vi "Vision Processing.vi"(4 "error in (no error)":errorcluster, 6 "CameraDevRef":T1) -> ()   [LabVIEW 2011]
uses:
  <vilib>/Rock Robotics/WPI/Camera/WPI_CameraDevRef.ctl
  Robot Global Data.vi
  <vilib>/vision/NI_Vision_Development_Module.lvlib
panel:
  in  "Run Calculations":bool
  out "Raw Turret":dbl
  out "Target X Coord":dbl
  out "Target Distance":dbl
  out "Target Y Coord":dbl
  out "Distance Array":dbl[](array[numeric])
  in  "Scaler":dbl=0.85
  in  "Lower Speed Limit":dbl=0.05
  out "Number of Rectangles Visible":dbl
  out "Y Position Array":dbl[](array[numeric])
  out "X Position Array":dbl[](array[numeric])
  in  "View":bool
  out "Target Info":T2(array[cluster])
  in  "Area Size Limit":i32=444
  in  "Particle Count Limit":i32=8
  in  "Score Limits":T3={"Rect Coverage"=76.0, "Aspect Ratio"=40.0, "X Edge Strength"=40.0, "Y Edge Strength"=60.0}
  in  "Processing":enum32{"Color", "Intensity", "Intensity Open"}(tab)=enum."Intensity Open"
  in  "Luminance":i32=255
  in  "Saturation":i32=255
  in  "Hue":i32(knob)=65 scale=0.0..255.0
  in  "Margins":cluster{"Hue":i32, "Sat":i32, "Lum":i32}={"Hue"=20, "Sat"=27, "Lum"=30} {"Sat" scale=0.0..40.0; "Lum" scale=0.0..40.0; "Hue" scale=0.0..40.0}
  in  "Range":cluster{"Lower value":sgl, "Upper value":sgl}={"Lower value"=150.0, "Upper value"=255.0} {"Lower value" scale=0.0..255.0; "Upper value" scale=0.0..255.0}
  in  "Range":cluster{"Lower value":sgl, "Upper value":sgl}={"Lower value"=123.804344, "Upper value"=255.0} {"Lower value" scale=0.0..255.0; "Upper value" scale=0.0..255.0}
  in  "View":bool
  out "Processed Image":T4(plugin-control)
  out "Original Image":T4(plugin-control)
  # "Instructions:\nProcessing the reflective tape that is illuminated by a ring light can be based\non color or light intensity.\nParticles within the image are scored by rectangle coverage, aspect ratio, and\nfor being hollow with a bold edge. A particle is considered a target if all scores\nare above the score limits. Particles can be annotated -- surrounded by\na rectangle and scores drawn to the left .\nTo control the number of particles being scored, use the count limit and the size\nlimit."
  # "To debug, Enable using the View button.\nFor color processing, you can click in the image to select the color for processing."
  # "Enable by clicking the View button.\nGreen scores are above the limit, orange are below. Inner/outer rect\nindicates all passed."
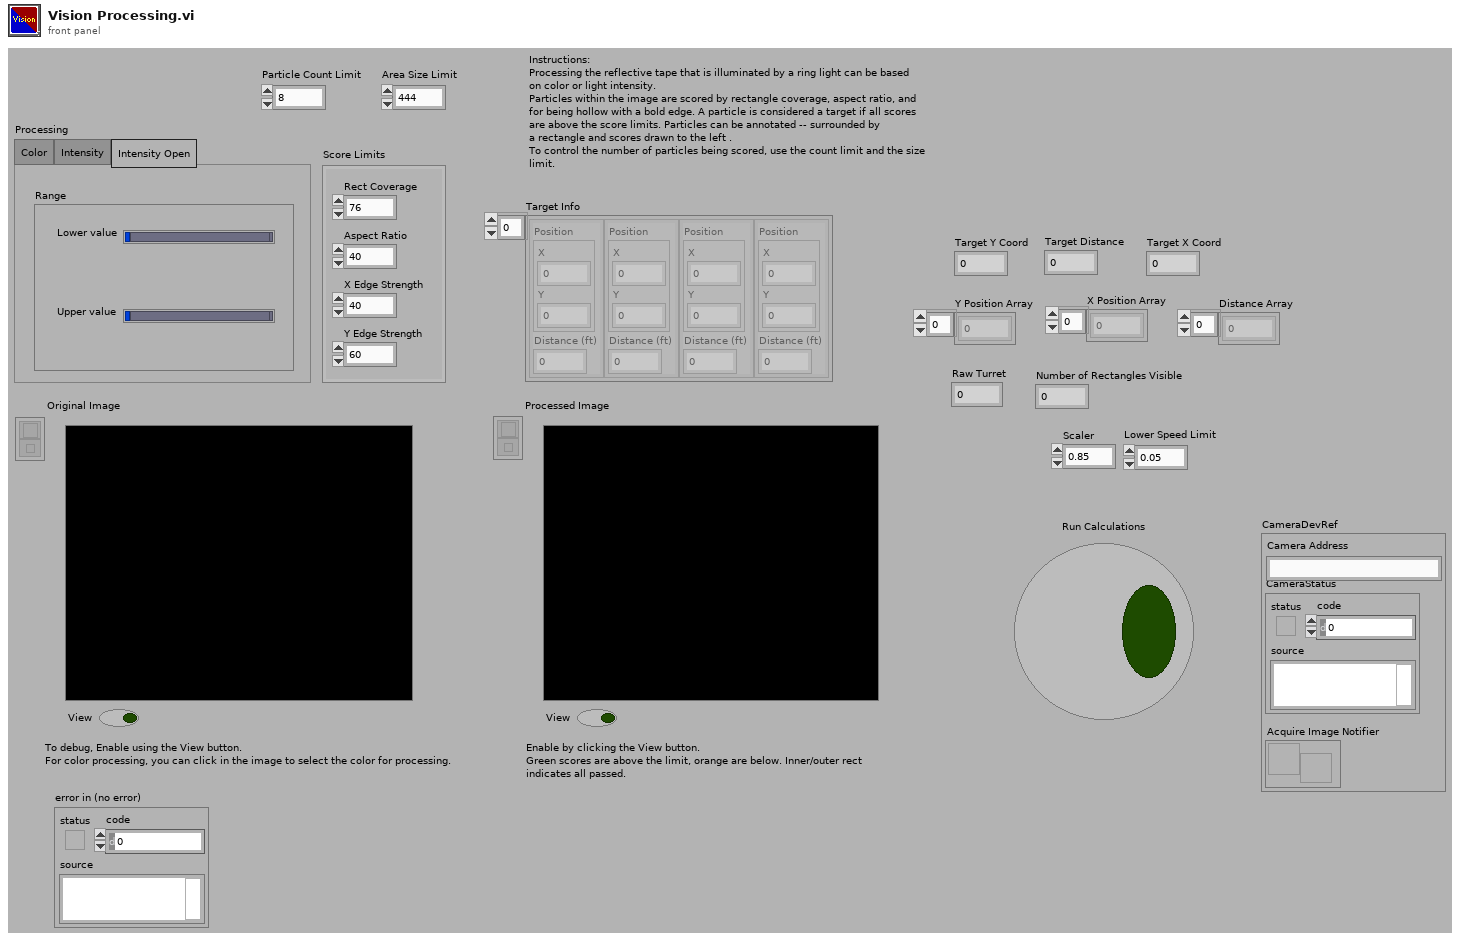
[diagram p1: front panel]
types:
  T1 = typedef "WPI_CameraDevRef.ctl" = cluster{"Camera Address":string, "CameraStatus":errorcluster, "Acquire Image Notifier":refnum<notifier>}
  T2 = cluster{"Position":cluster{"X":dbl, "Y":dbl}, "Distance (ft)":dbl}[]
  T3 = cluster{"Rect Coverage":dbl, "Aspect Ratio":dbl, "X Edge Strength":dbl, "Y Edge Strength":dbl}
  T4 = typedef "IMAQ Image.ctl" = refnum<image>
  T5 = typedef "Image Type" = u32
  T6 = enum32{"AutoM", "Close", "Dilate", "Erode", "Gradient", "Gradient out", "Gradient in", "Hit miss", "Open", "PClose", "POpen", "Thick", "Thin"}
  T7 = typedef "WPI_CameraImageSize.ctl" = enum16{"640x480", "320x240", "160x120"}
  T8 = cluster{"fps":i32, "compression":i32, "Image Size":T7}
  T9 = cluster{cluster{"Left":dbl, "Top":dbl, "Right":dbl, "Bottom":dbl}, dbl[]}[]
  T10 = cluster{"Left":dbl, "Top":dbl, "Right":dbl, "Bottom":dbl}
  T11 = cluster{"Target Center (-1 to 1)":cluster{"X":dbl, "Y":dbl}, "Distance (ft)":dbl}
  T12 = cluster{"Target Center (-1 to 1)":cluster{"X":dbl, "Y":dbl}, "Distance (ft)":dbl}[]
  T13 = typedef "WPI_JoystickDevRef.ctl" = cluster{"Device":T14}
  T14 = typedef "WPI_JoystickDeviceEnum.ctl" = enum16{"USB 1", "USB 2", "USB 3", "USB 4", "Kinect 1", "Kinect 2"}
  T15 = typedef "WPI_JoystickButtonState.ctl" = cluster{"Button 1":bool, "Button 2":bool, "Button 3":bool, "Button 4":bool, "Button 5":bool, "Button 6":bool, "Button 7":bool, "Button 8":bool, "Button 9":bool, "Button 10":bool, "Button 11":bool, "Button 12":bool}
  T16 = cluster{"axis 1 (x)":dbl, "axis 2 (y)":dbl, "axis 3 (throttle)":dbl, "axis 4":dbl, "axis 5":dbl, "axis 6":dbl}
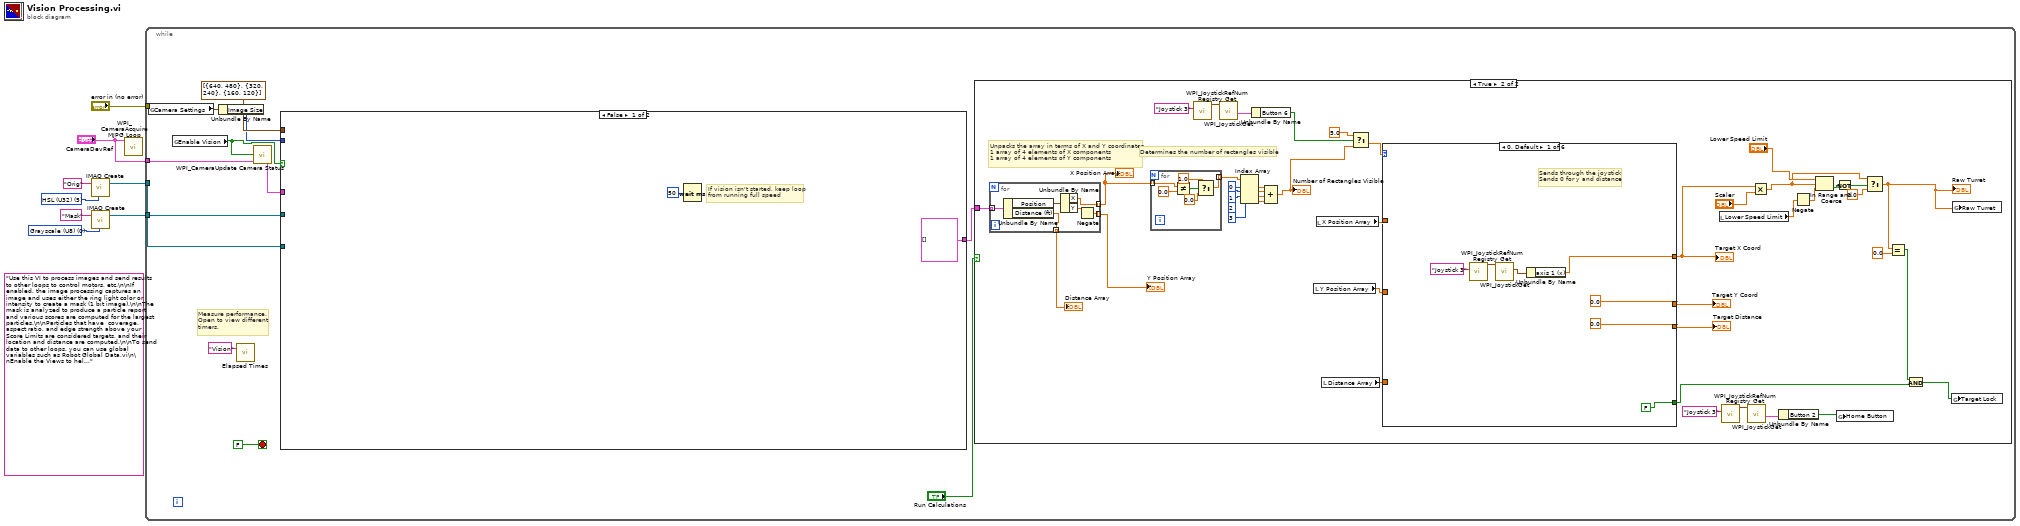
[diagram p0: block diagram]
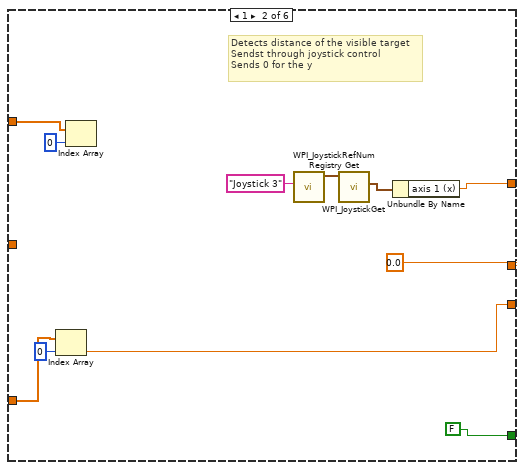
[diagram p3: hidden frame]
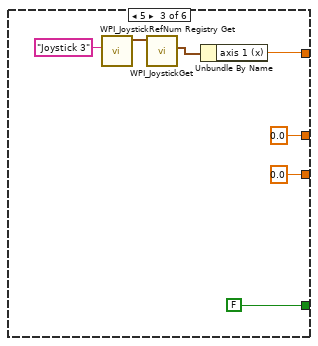
[diagram p4: hidden frame]
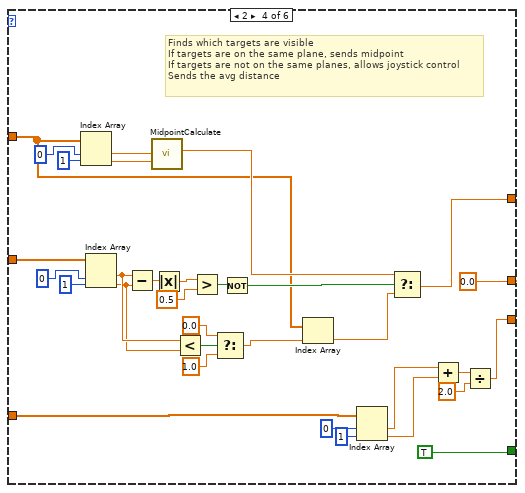
[diagram p5: hidden frame]
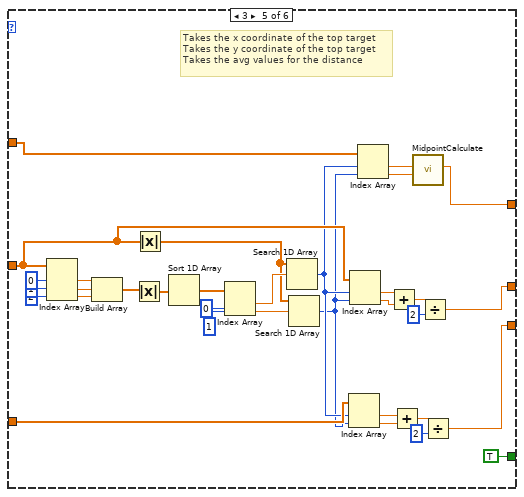
[diagram p6: hidden frame]
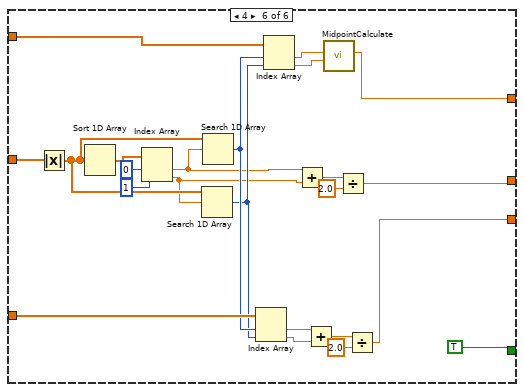
[diagram p7: hidden frame]
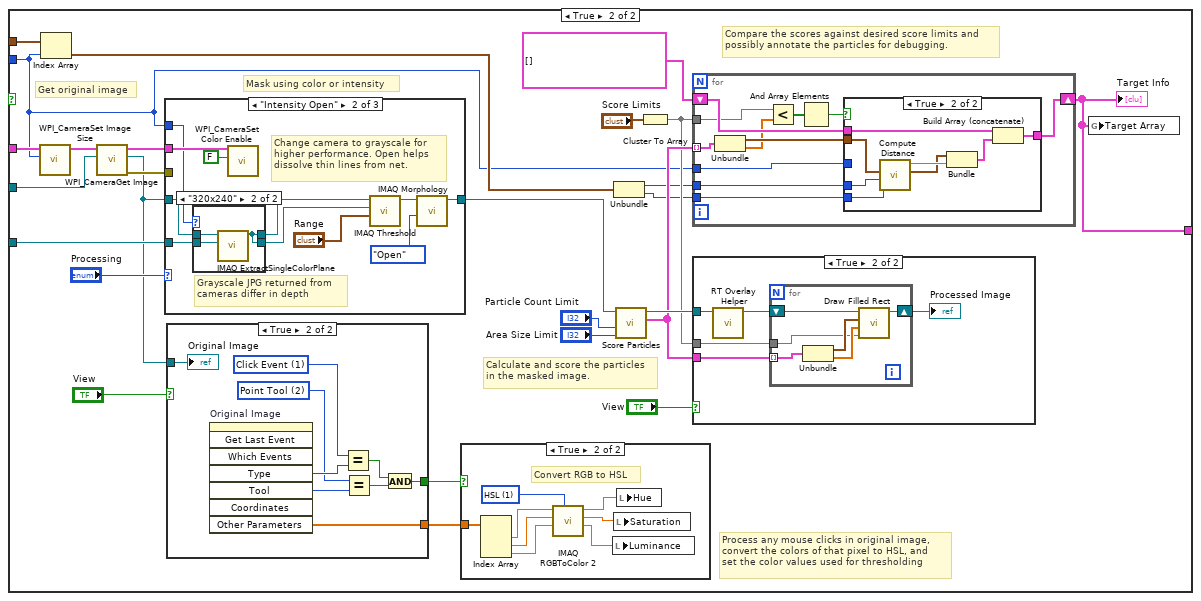
[diagram p8: hidden frame]
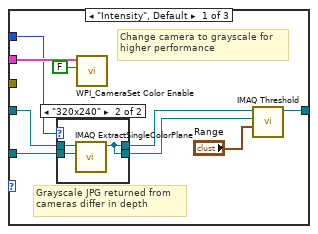
[diagram p10: hidden frame]
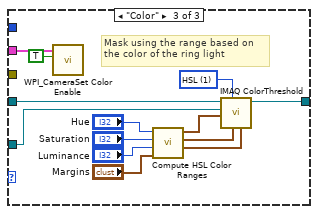
[diagram p13: hidden frame]
diagram:
  w3 = T5 0 items=["Grayscale (U8)", "Grayscale (I16)", "Grayscale (SGL)", "Complex (CSG)", "RGB (U32)", "HSL (U32)", "RGB (U64)", "Grayscale (U16)"] ("Image Type")
  (unwired) "Use this VI to process images and send results to other loops to control motors, etc.\n\nIf enabled, the image processing captures an image and uses either the ring light color or intensity to create a mask (1 bit image).\n\nThe mask is analyzed to produce a particle report and various scores are computed for the largest particles.\n\nParticles that have  coverage, aspect ratio, and edge strength above your Score Limits are considered targets, and their location and distance are computed.\n\nTo send data to other loops, you can use global variables such as Robot Global Data.vi\n\nEnable the Views to help debug color settings. Disable the View to speed up processing."
  w7 = T5 5 items=["Grayscale (U8)", "Grayscale (I16)", "Grayscale (SGL)", "Complex (CSG)", "RGB (U32)", "HSL (U32)", "RGB (U64)", "Grayscale (U16)"] ("Image Type")
  n1 = call "IMAQ Create"("Image Name"="Orig", "Image Type"=w7) -> ("New Image"=w6:T4)  [unwired: 2 in, 2 out]
  n2 = call "IMAQ Create"("Image Name"="Mask", "Image Type"=w3) -> ("New Image"=w1:T4)  [unwired: 2 in, 2 out]
  n3 = call <vilib>:"WPI_CameraAcquire MJPG Loop.vi"("CameraDevRef"="CameraDevRef") -> ()  [unwired: 11 in]
  n4 = while {
    tunnel: w6 -> [w19]
    tunnel: "CameraDevRef" -> [w18]
    tunnel: "error in (no error)" -> [_]
    tunnel: w1 -> [w14]
    stop <- FALSE stop-if-true
    # "Measure performance.\nOpen to view different\ntimers."
    n5 = global read "Robot Global Data.vi" "Camera Settings"() -> (w12:T8)
    n6 = global read "Robot Global Data.vi" "Enable Vision"() -> (w16:bool)
    n7 = Unbundle By Name(w12) -> ("Image Size"=w11:T7)
    n8 = call "Elapsed Times.vi"("Call Name"="Vision") -> ()  [unwired: 2 in, 1 out]
    n9 = call <vilib>:"WPI_CameraUpdate Camera Status.vi"("CameraDevRef In"=w18, "Enable Vision"=w16) -> ("CameraDevRef Out"=w17:T1)  [unwired: 3 in]
    n10 = case shown="False" w16 {
      tunnel: w19 -> [_ w207]
      tunnel: w17 -> [_ w203]
      tunnel: w14 -> [_ w194]
      tunnel: cluster{i32, i32}[] [{640, 480}, {320, 240}, {160, 120}] -> [_ w198]
      tunnel: w11 -> [_ w191]
      tunnel: [T2 [] w192] -> w10
      frame False {
        # "If vision isn't started, keep loop\nfrom running full speed"
        n11 = Wait (ms)(milliseconds to wait=u32 50) -> ()  [unwired: 1 out]
      }
      frame True {
        # "Compare the scores against desired score limits and\npossibly annotate the particles for debugging."
        # "Process any mouse clicks in original image,\nconvert the colors of that pixel to HSL, and\nset the color values used for thresholding"
        # "Calculate and score the particles\nin the masked image."
        # "Mask using color or intensity"
        # "Get original image"
        n12 = call <vilib>:"WPI_CameraSet Image Size.vi"("Image Size"=w191, "CameraDevRef"=w203) -> ("CameraDevRef Out"=w204:T1)  [unwired: 8 in, 1 out]
        n13 = Index Array(array=w198, index=w191) -> (element=w195:cluster{i32, i32})
        n14 = call <vilib>:"WPI_CameraGet Image.vi"("Image"=w207, "CameraDevRef"=w204) -> ("error out"=w205:errorcluster, "Image Out"=w193:T4, "CameraDevRef Out"=w206:T1)  [unwired: 7 in]
        n15 = case shown="\"Intensity Open\"" "Processing" {
          tunnel: w193 -> [w229 w241 w267]
          tunnel: [w232 w246 w266] -> w201
          tunnel: w206 -> [w230 w244 w257]
          tunnel: w205 -> [_ _ _]
          tunnel: w194 -> [w228 w242 w255]
          tunnel: w191 -> [w227 w243 _]
          frame "Intensity", Default {
            # "Grayscale JPG returned from\ncameras differ in depth"
            # "Change camera to grayscale for\nhigher performance"
            n16 = case shown="\"320x240\"" w227 {
              tunnel: w229 -> [w235 w238]
              tunnel: w228 -> [w234 w237]
              tunnel: [w235 w236] -> w226
              tunnel: [w234 w236] -> w225
              frame "640x480", Default {
              }
              frame "320x240" {
                n17 = call "IMAQ ExtractSingleColorPlane"("Image Dst"=w237, "Image Src"=w238) -> ("Image Dst Out"=w236:T4)  [unwired: 8 in, 1 out]
              }
            }
            n18 = call <vilib>:"WPI_CameraSet Color Enable.vi"("Color Enabled"=FALSE, "CameraDevRef"=w230) -> ()  [unwired: 8 in, 2 out]
            n19 = call "IMAQ Threshold"("Range"="Range", "Image Dst"=w225, "Image Src"=w226) -> ("Image Dst Out"=w232:T4)  [unwired: 3 in, 5 out]
          }
          frame "Intensity Open" {
            # "Grayscale JPG returned from\ncameras differ in depth"
            # "Change camera to grayscale for\nhigher performance. Open helps\ndissolve thin lines from net."
            n20 = case shown="\"320x240\"" w243 {
              tunnel: w241 -> [w251 w254]
              tunnel: w242 -> [w250 w253]
              tunnel: [w251 w252] -> w240
              tunnel: [w250 w252] -> w239
              frame "640x480", Default {
              }
              frame "320x240" {
                n21 = call "IMAQ ExtractSingleColorPlane"("Image Dst"=w253, "Image Src"=w254) -> ("Image Dst Out"=w252:T4)  [unwired: 8 in, 1 out]
              }
            }
            n22 = call <vilib>:"WPI_CameraSet Color Enable.vi"("Color Enabled"=FALSE, "CameraDevRef"=w244) -> ()  [unwired: 8 in, 2 out]
            n23 = call "IMAQ Threshold"("Range"="Range", "Image Dst"=w239, "Image Src"=w240) -> ("Image Dst Out"=w247:T4)  [unwired: 3 in, 5 out]
            n24 = call "IMAQ Morphology"("Operation"=T6."Open", "Image Src"=w247) -> ("Image Dst Out"=w246:T4)  [unwired: 8 in, 1 out]
          }
          frame "Color" {
            w265 = u16 1 items=["RGB", "HSL", "HSV", "HSI"] ("Color Mode")
            # "Mask using the range based on\nthe color of the ring light"
            n25 = call <vilib>:"WPI_CameraSet Color Enable.vi"("Color Enabled"=TRUE, "CameraDevRef"=w257) -> ()  [unwired: 8 in, 2 out]
            n26 = call "Compute HSL Color Ranges.vi"("Margins"="Margins", "Luminance"="Luminance", "Saturation"="Saturation", "Hue"="Hue") -> ("Lum Range"=w262:cluster{i32, i32}, "Sat Range"=w263:cluster{i32, i32}, "Hue Range"=w264:cluster{i32, i32})  [unwired: 5 in]
            n27 = call "IMAQ ColorThreshold"("Blue or Luma or Val or Inten Range"=w262, "Green or Sat Range"=w263, "Color Mode"=w265, "Red or Hue Range"=w264, "Image Dst"=w255, "Image Src"=w267) -> ("Image Dst Out"=w266:T4)  [unwired: 4 in, 1 out]
          }
        }
        n28 = case shown="True" "View" {
          tunnel: w193 -> [_ w287]
          tunnel: [_ w282] -> w200
          tunnel: [_ w279] -> w199
          frame False {
          }
          frame True {
            w280 = 2 items=["None", "Selection Tool", "Point Tool", "Line Tool", "Rectangle Tool", "Oval Tool", "Polygon Tool", "ClosedFreehandTool", "Annulus Tool", "Rotated Rectangle Tool", "Zoom Tool", "Pan Tool", "Polyline Tool", "Freehand Tool"] ("Tool")
            w281 = 1 items=["No Event"=0, "Click Event"=1, "Draw Event"=2, "Size Event"=4, "Scroll Event"=5, "Double Click Event"=8] ("Type")
            n29 = invoke on="Original Image" class="ImageControl" method="Get Last Event"() -> ("Type"=w283:i32, "Tool"=w286:i32, "Other Parameters"=w279:sgl[])  [unwired: 8 in, 5 out]
            n30 = Equal?(x=w281, y=w283) -> (x = y?=w284:bool)
            n31 = Equal?(x=w280, y=w286) -> (x = y?=w285:bool)
            n32 = And(x=w284, y=w285) -> (x .and. y?=w282:bool)
            "Original Image" <- w287
          }
        }
        n33 = case shown="True" w200 {
          tunnel: w199 -> [_ w224]
          frame False {
          }
          frame True {
            w223 = u16 1 items=["RGB", "HSL", "HSV", "HSI", "CIE L*a*b*", "CIE XYZ"] ("Color Mode")
            # "Convert RGB to HSL"
            n34 = Index Array(array=w224) -> (element #1=w222:sgl, element #2=w220:sgl, element #3=w218:sgl)  [unwired: 3 in]
            n35 = call "IMAQ RGBToColor 2"("Color Mode"=w223, "Blue value"=w218, "Green value"=w220, "Red value"=w222) -> ("Blue or Luma or Val or Inten or Z or b*value"=w217:dbl, "Green or Sat or Y or a* value"=w219:dbl, "Red or Hue or X or L* value"=w221:dbl)  [unwired: 4 in, 1 out]
            n36 = local write "Luminance"(w217) -> ()
            n37 = local write "Saturation"(w219) -> ()
            n38 = local write "Hue"(w221) -> ()
          }
        }
        n39 = Unbundle(w195) -> (w197:i32, w196:i32)
        n40 = call "Score Particles.vi"("Area Size Limit"="Area Size Limit", "Particle Count Limit"="Particle Count Limit", "Image Refnum in"=w201) -> ("Scored Particle Info"=w212:T9, "Image Refnum out"=w215:T4)  [unwired: 7 in]
        n41 = Cluster To Array(cluster="Score Limits") -> (array=w210:dbl[])
        n42 = for {
          shift-right: [w297] -> w192
          shift-left: T2 [] -> [w298]
          tunnel: w197 -> [w296]
          tunnel: w212 -> [w294] mode=indexing
          tunnel: w210 -> [w289]
          tunnel: w191 -> [w293]
          tunnel: w196 -> [w288]
          n43 = Unbundle(w294) -> (w295:T10, w290:dbl[])
          n44 = Less?(x=w289, y=w290) -> (x < y?=w292:bool[])
          n45 = And Array Elements(Boolean array=w292) -> (logical AND=w291:bool)
          n46 = case shown="True" w291 {
            tunnel: w298 -> [w299 w307]
            tunnel: [w299 w306] -> w297
            tunnel: w295 -> [_ w302]
            tunnel: w296 -> [_ w304]
            tunnel: w293 -> [_ _]
            tunnel: w288 -> [_ w301]
            frame False {
            }
            frame True {
              n47 = call "Compute Distance.vi"("Y Image Resolution"=w301, "X Image Resolution"=w304, "Bounding Box"=w302) -> ("Target Center (-1 to 1)"=w300:cluster{"X":dbl, "Y":dbl}, "Distance (ft)"=w303:dbl)  [unwired: 7 in]
              n48 = Bundle("Target Center (-1 to 1)"=w300, "Distance (ft)"=w303) -> (w305:T11)  [unwired: 1 in]
              n49 = Build Array (concatenate)(w307, w305) -> (w306:T12)
            }
          }
        }
        "Target Info" <- w192
        n50 = case shown="True" "View" {
          tunnel: w215 -> [_ w269]
          tunnel: w212 -> [_ w271]
          tunnel: w210 -> [_ w270]
          frame False {
          }
          frame True {
            n51 = call "RT Overlay Helper.vi"("Refnum in"=w269) -> ("Refnum out"=w272:T4)  [unwired: 10 in]
            n52 = for {
              shift-right: [w277] -> w268
              shift-left: w272 -> [w278]
              tunnel: w271 -> [w274] mode=indexing
              tunnel: w270 -> [w273]
              n53 = Unbundle(w274) -> (w275:T10, w276:dbl[])
              n54 = call "Draw Filled Rect.vi"("Limits"=w273, "Scores"=w276, "Bounding Box"=w275, "image in"=w278) -> ("image out"=w277:T4)  [unwired: 7 in]
            }
            "Processed Image" <- w268
          }
        }
        n55 = global write "Robot Global Data.vi" "Target Array"(w192) -> ()
      }
    }
    n56 = case shown="True" "Run Calculations" {
      tunnel: w10 -> [_ w35]
      frame False {
      }
      frame True {
        # "Determines the number of rectangles visible"
        # "Unpacks the array in terms of X and Y coordinates\n1 array of 4 elements of X components\n1 array of 4 elements of Y components"
        n57 = for {
          tunnel: [w186] -> w36 mode=indexing
          tunnel: [w187] -> w46 mode=indexing
          tunnel: w35 -> [w184] mode=indexing
          tunnel: [w183] -> w55 mode=indexing
          n58 = Unbundle By Name(w184) -> ("Position"=w188:cluster{"X":dbl, "Y":dbl}, "Distance (ft)"=w183:dbl)
          n59 = Unbundle By Name(w188) -> ("X"=w187:dbl, "Y"=w185:dbl)
          n60 = Negate(x=w185) -> (-x=w186:dbl)
        }
        "X Position Array" <- w46
        "Y Position Array" <- w36
        "Distance Array" <- w55
        n61 = for {
          tunnel: w46 -> [w68] mode=indexing
          tunnel: [w64] -> w45 mode=indexing
          n62 = Not Equal?(x=w68, y=0.0) -> (x != y?=w67:bool)
          n63 = Select(t=1.0, s=w67, f=0.0) -> (s? t:f=w64:dbl)
        }
        n64 = call <vilib>:"WPI_JoystickRefNum Registry Get.vi"("refnum name"="Joystick 3") -> ("JoystickDevRef"=w24:T13)  [unwired: 9 in, 1 out]
        n65 = call <vilib>:"WPI_JoystickGet.vi"("JoystickDevRef"=w24) -> ("Buttons"=w22:T15)  [unwired: 4 in, 2 out]
        n66 = Index Array(array=w45, index #1=0 ("index"), index #2=1 ("index"), index #3=2 ("index"), index #4=3 ("index")) -> (element #1=w43:dbl, element #2=w44:dbl, element #3=w42:dbl, element #4=w41:dbl)
        n67 = Unbundle By Name(w22) -> ("Button 6"=w21:bool)
        n68 = Compound Arithmetic op=ADD(w43, w44, w42, w41) -> (w34:dbl)
        "Number of Rectangles Visible" <- w34
        n69 = local read "Y Position Array"() -> (w59:dbl[])
        n70 = local read "X Position Array"() -> (w47:dbl[])
        n71 = local read "Distance Array"() -> (w60:dbl[])
        n72 = Select(t=5.0, s=w21, f=w34) -> (s? t:f=w62:dbl)
        n73 = case shown="0, Default" w62 {
          tunnel: w47 -> [_ w82 _ w97 w143 w176]
          tunnel: [w70 w77 w88 w115 w140 w166] -> w58
          tunnel: [0.0 ("X") 0.0 ("X") 0.0 ("X") 0.0 ("X") w144 w165] -> w56
          tunnel: [0.0 ("X") w85 0.0 ("X") w108 w128 w160] -> w57
          tunnel: w59 -> [_ _ _ w124 w136 w181]
          tunnel: w60 -> [_ w87 _ w107 w131 w175]
          tunnel: [FALSE FALSE FALSE TRUE TRUE TRUE] -> w31
          frame 0, Default {
            # "Sends through the joystick\nSends 0 for y and distance"
            n74 = call <vilib>:"WPI_JoystickRefNum Registry Get.vi"("refnum name"="Joystick 3") -> ("JoystickDevRef"=w73:T13)  [unwired: 9 in, 1 out]
            n75 = call <vilib>:"WPI_JoystickGet.vi"("JoystickDevRef"=w73) -> ("Axes"=w71:T16)  [unwired: 4 in, 2 out]
            n76 = Unbundle By Name(w71) -> ("axis 1 (x)"=w70:dbl)
          }
          frame 1 {
            # "Detects distance of the visible target\nSendst through joystick control\nSends 0 for the y"
            n77 = Index Array(array=w87, index=0) -> (element=w85:dbl)
            n78 = Index Array(array=w82, index=0) -> ()  [unwired: 1 out]
            n79 = call <vilib>:"WPI_JoystickRefNum Registry Get.vi"("refnum name"="Joystick 3") -> ("JoystickDevRef"=w80:T13)  [unwired: 9 in, 1 out]
            n80 = call <vilib>:"WPI_JoystickGet.vi"("JoystickDevRef"=w80) -> ("Axes"=w78:T16)  [unwired: 4 in, 2 out]
            n81 = Unbundle By Name(w78) -> ("axis 1 (x)"=w77:dbl)
          }
          frame 5 {
            n82 = call <vilib>:"WPI_JoystickRefNum Registry Get.vi"("refnum name"="Joystick 3") -> ("JoystickDevRef"=w91:T13)  [unwired: 9 in, 1 out]
            n83 = call <vilib>:"WPI_JoystickGet.vi"("JoystickDevRef"=w91) -> ("Axes"=w89:T16)  [unwired: 4 in, 2 out]
            n84 = Unbundle By Name(w89) -> ("axis 1 (x)"=w88:dbl)
          }
          frame 2 {
            # "Finds which targets are visible\nIf targets are on the same plane, sends midpoint\nIf targets are not on the same planes, allows joystick control\nSends the avg distance"
            n85 = Index Array(array=w97, index #1=0 ("index"), index #2=1 ("index")) -> (element #1=w113:dbl, element #2=w112:dbl)
            n86 = Index Array(array=w124, index #1=0 ("index"), index #2=1 ("index")) -> (element #1=w103:dbl, element #2=w102:dbl)
            n87 = Subtract(x=w103, y=w102) -> (x-y=w121:dbl)
            n88 = call "MidpointCalculate.vi"("X2"=w112, "X1"=w113) -> ("Midpoint"=w116:dbl)  [unwired: 9 in]
            n89 = Absolute Value(x=w121) -> (abs(x)=w120:dbl)
            n90 = Less?(x=w103, y=w102) -> (x < y?=w101:bool)
            n91 = Greater?(x=w120, y=0.5) -> (0:w117:bool)
            n92 = Select(t=0.0, s=w101, f=1.0) -> (s? t:f=w98:dbl)
            n93 = Not(x=w117) -> (.not. x?=w118:bool)
            n94 = Index Array(array=w97, index=w98) -> (element=w96:dbl)
            n95 = Index Array(array=w107, index #1=0 ("index"), index #2=1 ("index")) -> (element #1=w106:dbl, element #2=w105:dbl)
            n96 = Select(t=w116, s=w118, f=w96) -> (s? t:f=w115:dbl)
            n97 = Add(x=w106, y=w105) -> (x+y=w111:dbl)
            n98 = Divide(x=w111, y=2.0) -> (x/y=w108:dbl)
          }
          frame 3 {
            # "Takes the x coordinate of the top target\nTakes the y coordinate of the top target\nTakes the avg values for the distance"
            n99 = Index Array(array=w136, index #1=0 ("index"), index #2=1 ("index"), index #3=2 ("index")) -> (element #1=w156:dbl, element #2=w155:dbl, element #3=w154:dbl)
            n100 = Build Array(w156, w155, w154) -> (w153:dbl[])
            n101 = Absolute Value(x=w153) -> (abs(x)=w147:dbl[])
            n102 = Absolute Value(x=w136) -> (abs(x)=w139:dbl[])
            n103 = Sort 1D Array(array=w147) -> (sorted array=w152:dbl[])
            n104 = Index Array(array=w152, index #1=0 ("index"), index #2=1 ("index")) -> (element #1=w148:dbl, element #2=w149:dbl)
            n105 = Search 1D Array(1D array=w139, element=w148) -> (index of element=w130:i32)  [unwired: 1 in]
            n106 = Search 1D Array(1D array=w139, element=w149) -> (index of element=w129:i32)  [unwired: 1 in]
            n107 = Index Array(array=w131, index #1=w130, index #2=w129) -> (element #1=w133:dbl, element #2=w132:dbl)
            n108 = Index Array(array=w136, index #1=w130, index #2=w129) -> (element #1=w138:dbl, element #2=w137:dbl)
            n109 = Index Array(array=w143, index #1=w130, index #2=w129) -> (element #1=w142:dbl, element #2=w141:dbl)
            n110 = Add(x=w138, y=w137) -> (x+y=w146:dbl)
            n111 = Add(x=w133, y=w132) -> (x+y=w134:dbl)
            n112 = call "MidpointCalculate.vi"("X2"=w141, "X1"=w142) -> ("Midpoint"=w140:dbl)  [unwired: 9 in]
            n113 = Divide(x=w146, y=2) -> (x/y=w144:dbl)
            n114 = Divide(x=w134, y=2) -> (x/y=w128:dbl)
          }
          frame 4 {
            n115 = Absolute Value(x=w181) -> (abs(x)=w177:dbl[])
            n116 = Sort 1D Array(array=w177) -> (sorted array=w180:dbl[])
            n117 = Index Array(array=w180, index #1=0 ("index"), index #2=1 ("index")) -> (element #1=w172:dbl, element #2=w171:dbl)
            n118 = Search 1D Array(1D array=w177, element=w171) -> (index of element=w173:i32)  [unwired: 1 in]
            n119 = Search 1D Array(1D array=w177, element=w172) -> (index of element=w174:i32)  [unwired: 1 in]
            n120 = Index Array(array=w175, index #1=w174, index #2=w173) -> (element #1=w162:dbl, element #2=w161:dbl)
            n121 = Index Array(array=w176, index #1=w174, index #2=w173) -> (element #1=w168:dbl, element #2=w167:dbl)
            n122 = Add(x=w172, y=w171) -> (x+y=w170:dbl)
            n123 = Add(x=w162, y=w161) -> (x+y=w163:dbl)
            n124 = call "MidpointCalculate.vi"("X2"=w167, "X1"=w168) -> ("Midpoint"=w166:dbl)  [unwired: 9 in]
            n125 = Divide(x=w170, y=2.0) -> (x/y=w165:dbl)
            n126 = Divide(x=w163, y=2.0) -> (x/y=w160:dbl)
          }
        }
        "Target Y Coord" <- w56
        "Target Distance" <- w57
        "Target X Coord" <- w58
        n127 = local read "Lower Speed Limit"() -> (w49:dbl)
        n128 = call <vilib>:"WPI_JoystickRefNum Registry Get.vi"("refnum name"="Joystick 3") -> ("JoystickDevRef"=w28:T13)  [unwired: 9 in, 1 out]
        n129 = call <vilib>:"WPI_JoystickGet.vi"("JoystickDevRef"=w28) -> ("Buttons"=w26:T15)  [unwired: 4 in, 2 out]
        n130 = Multiply(x=w58, y="Scaler") -> (x*y=w54:dbl)
        n131 = Unbundle By Name(w26) -> ("Button 2"=w25:bool)
        n132 = Negate(x=w49) -> (-x=w50:dbl)
        n133 = In Range and Coerce(upper limit="Lower Speed Limit", x=w54, lower limit=w50) -> (In Range?=w51:bool)  [unwired: 1 out]
        n134 = Not(x=w51) -> (.not. x?=w52:bool)
        n135 = global write "Robot Global Data.vi" "Home Button"(w25) -> ()
        n136 = Select(t=w54, s=w52, f=0.0) -> (s? t:f=w33:dbl)
        "Raw Turret" <- w33
        n137 = Equal?(x=w33, y=0.0) -> (x = y?=w30:bool)
        n138 = And(x=w30, y=w31) -> (x .and. y?=w29:bool)
        n139 = global write "Robot Global Data.vi" "Target Lock"(w29) -> ()
        n140 = global write "Robot Global Data.vi" "Raw Turret"(w33) -> ()
      }
    }
  }
